vi "NameToDICOMFormat.vi"(11 "Name In":string) -> (3 "Name Out":string)   [LabVIEW 2013, in "main.lvlib"]
uses:
  main.lvlib
panel:
  in  "error in (no error)":errorcluster
  out "error out":errorcluster
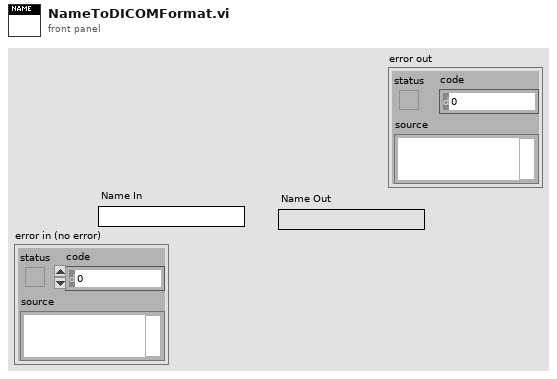
[diagram p1: front panel]
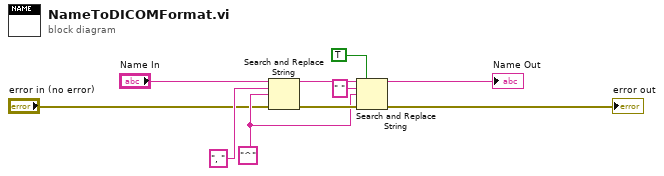
[diagram p0: block diagram]
diagram:
  w4 = "^" ("replace string (\"\")")
  n1 = Search and Replace String(input string="Name In", search string=", ", replace string=w4, error in="error in (no error)") -> (result string=w8:string, error out=w7:errorcluster)  [unwired: 4 in, 2 out]
  n2 = Search and Replace String(replace all?=TRUE ("replace all? (F)"), input string=w8, search string=" ", replace string=w4, error in=w7) -> (result string=→"Name Out":string, error out=→"error out":errorcluster)  [unwired: 3 in, 2 out]
